vi "DAQmx连续波形输出.vi"() -> ()   [LabVIEW 2010]
doc: "I. Description:\nThis example demonstrates how to continuously output a waveform using an internal sample clock. The update rate can be changed while the continuous generation is taking place.\n\nII. Instructions for Running:\n1. Select the Physical Channel to correspond to where your signal is output on the DAQ device.\n2. Enter the Minimum and Maximum Voltage ranges.\n3. Specify the Desired Frequency of the output Waveform. This control can be modified while the generation is taking place.\n4. Enter the Waveform Information. See the documentation of the Waveform Buffer Generation SubVI for information on each parameter.\n\nIII. Block Diagram Steps:\n1. Create an Analog Output Voltage Channel\n2. Call the DAQmx (Sample Clock) VI which sets the sample clock rate based on the rate calculated in the Waveform Buffer Generation subVI. Additionally, set the sample mode to Continuous.\n3. Write the waveform to the output buffer.\n4. Call the Start VI.\n5. Obtain the current value of the Desired Frequency control using a local variable.\n6. Set the sample clock rate to the current desired frequency value using the Waveform Buffer Generation subVI. The Loop runs continuously until user presses the Stop button or an error occurs. Check for errors every 100 ms using the Is Task Done? VI\n7. Call the Clear Task VI to clear the Task.\n8. Use the popup dialog box to display an error or warning if any.\n\nIV. I/O Connections Overview:\nMake sure your signal output terminal matches the Physical Channel I/O Control. For further connection information, refer to your hardware reference manual."
uses:
  <vilib>/Utility/error.llb/DialogType.ctl
  <vilib>/DAQmx/write.llb/DAQmx Write (Analog 1D Wfm NChan NSamp).vi
  <vilib>/DAQmx/create/channels.llb/DAQmx Create Channel (AO-Voltage-Basic).vi
  <vilib>/DAQmx/configure/timing.llb/DAQmx Timing (Sample Clock).vi
  <vilib>/daqmx/miscellaneous.llb/DAQmx Fill In Error Info.vi
  C:/Program Files/National Instruments/LabVIEW 2010/resource/objmgr/daqmx.rc
panel:
  in  "Cycles per Buffer":i32=5
  in  "Waveform Type":T1(ring)
  in  "Desired Frequency":dbl=1000.0 format="%.2f"
  in  "Samples per Buffer":dbl=250.0
  in  "Amplitude":dbl=2.0 format="%0.2p"
  out "输出波形":waveform(dbl)[](graph) caption="Output Waveform"
  in  "Physical Channels":tag="Dev1/ao0"
  in  "Minimum Value":dbl=-10.0 format="%0.2f"
  in  "Maximum Value":dbl=10.0 format="%0.2f"
  in  "stop":bool
  # "For instructions, select Help>>Show Context Help"
  # "Channel Parameters"
  # "Timing Parameters"
  # "Waveform Information"
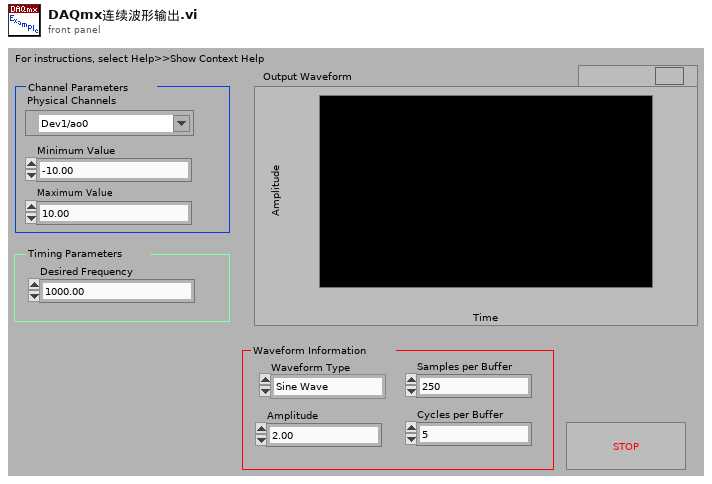
[diagram p1: front panel]
types:
  T1 = enum16{"Sine Wave", "Triangle Wave", "Square Wave", "Sawtooth Wave"}
  T2 = typedef "DialogType.ctl" = u16
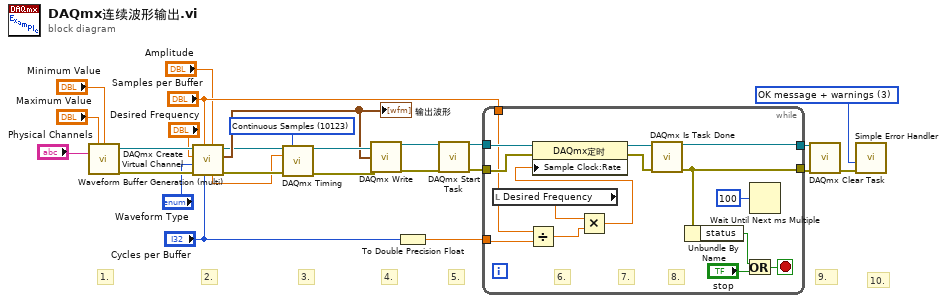
[diagram p0: block diagram]
diagram:
  w17 = T2 3 items=["no dialog", "OK message", "continue or stop message", "OK message + warnings", "continue/stop + warnings"] ("type of dialog (OK msg:1)")
  w25 = 10123 items=["Finite Samples"=10178, "Continuous Samples"=10123] ("sample mode")
  # "10."
  # "9."
  # "5."
  # "3."
  # "4."
  # "2."
  # "1."
  n1 = call-poly <vilib>:"DAQmx Create Virtual Channel.vi"("maximum value"="Maximum Value", "minimum value"="Minimum Value", "physical channels"="Physical Channels") -> ("task out"=w11:refnum<k21>, "error out"=w8:errorcluster)  [unwired: 11 in]
  n2 = call "Waveform Buffer Generation (multi).vi"("Amplitude"="Amplitude", "Cycles per Buffer"="Cycles per Buffer", "Samples per Buffer"="Samples per Buffer", "error in (no error)"=w8, "Waveform Type"="Waveform Type", "Desired Frequency"="Desired Frequency", "task/channels in"=w11) -> ("error out"=w9:errorcluster, "Waveform"=w15:waveform(dbl)[], "task out"=w10:refnum<k21>, "Resulting Sample Clock Rate"=w5:dbl)  [unwired: 1 out]
  "输出波形" <- w15
  n3 = call-poly <vilib>:"DAQmx Timing.vi"("task/channels in"=w10, "sample mode"=w25, "rate"=w5, "error in"=w9) -> ("task out"=w18:refnum<k21>, "error out"=w12:errorcluster)  [unwired: 10 in]
  n4 = call-poly <vilib>:"DAQmx Write.vi"("task/channels in"=w18, "data"=w15, "error in"=w12) -> ("task out"=w22:refnum<k21>, "error out"=w21:errorcluster)  [unwired: 10 in, 1 out]
  n5 = To Double Precision Float(number="Cycles per Buffer") -> (double precision float=w1:dbl)
  n6 = call <vilib>:"DAQmx Start Task.vi"("task/channels in"=w22, "error in"=w21) -> ("task out"=w26:refnum<k21>, "error out"=w20:errorcluster)  [unwired: 12 in]
  n7 = while {
    tunnel: w26 -> [w31]
    tunnel: [w36] -> w14
    tunnel: w20 -> [w30]
    tunnel: [w37] -> w13
    tunnel: "Samples per Buffer" -> [w29]
    tunnel: w1 -> [w34]
    stop <- w41 stop-if-true
    # "8."
    # "7."
    # "6."
    n8 = local read "Desired Frequency"() -> (w35:dbl)
    n9 = Divide(x=w29, y=w34) -> (x/y=w28:dbl)
    n10 = Multiply(x=w35, y=w28) -> (x*y=w27:dbl)
    n11 = property class="DAQmx定时"(reference=w31, error in=w30, "Sample Clock:Rate"=w27) -> (reference out=w33:refnum<k21>, error out=w32:errorcluster)
    n12 = call <vilib>:"DAQmx Is Task Done.vi"("task/channels in"=w33, "error in"=w32) -> ("task out"=w36:refnum<k21>, "error out"=w37:errorcluster)  [unwired: 11 in, 1 out]
    n13 = Unbundle By Name(w37) -> ("status"=w39:bool)
    n14 = Or(x=w39, y="stop") -> (x .or. y?=w41:bool)
    n15 = Wait Until Next ms Multiple(millisecond multiple=u32 100) -> ()  [unwired: 1 out]
  }
  n16 = call <vilib>:"DAQmx Clear Task.vi"("task in"=w14, "error in"=w13) -> ("error out"=w16:errorcluster)  [unwired: 13 in]
  n17 = call <vilib>:"Simple Error Handler.vi"("type of dialog (OK msg:1)"=w17, "error in (no error)"=w16) -> ()  [unwired: 3 in, 5 out]
